vi "Update-PV.vi"(8 "Error In":errorcluster, 10 "PV":refnum<class "PV.lvclass">, 11 "CS++GUIActor in":refnum<class "CS++GUIActor.lvclass">) -> (0 "Error Out":errorcluster, 3 "CS++GUIActor out":refnum<class "CS++GUIActor.lvclass">)   [LabVIEW 2015, in "CS++GUIActor.lvlib" / "CS++GUIActor.lvclass"]
doc: "Send PV-Event to Actore Core.vi"
uses:
  CS++GUIActor.lvclass
  Classes/CS++ProcessVariables/ProcessVariable/PV.lvclass
  CS++GUIActor.lvclass/CS++GUIActor.ctl
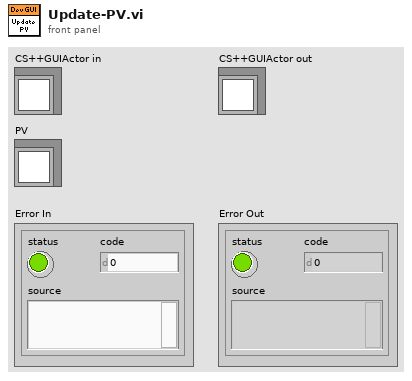
[diagram p1: front panel]
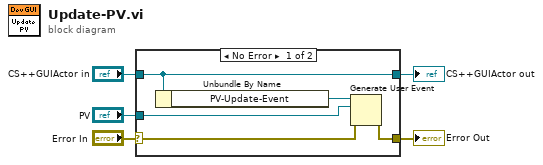
[diagram p0: block diagram]
diagram:
  n1 = case shown="No Error" "Error In" {
    selector: "Error In" -> [w7 w12]
    tunnel: [w6 w12] -> w4
    tunnel: [w10 w11] -> w2
    tunnel: "CS++GUIActor in" -> [w10 w11]
    tunnel: "PV" -> [w8 _]
    frame No Error {
      n2 = Unbundle By Name(w10) -> ("PV-Update-Event"=w9:refnum<user-event>)
      n3 = Generate User Event(user event=w9, event data cluster=w8, error in=w7) -> (error out=w6:errorcluster)  [unwired: 1 in, 1 out]
    }
    frame Error {
    }
  }
  "Error Out" <- w4
  "CS++GUIActor out" <- w2
